vi "example_GProgramUploadFile.vi"() -> ()   [LabVIEW 2020]
uses:
  <vilib>/Galil/resources/gclib/gclib.lvlib
  <vilib>/Galil/resources/gclibo/gclibo.lvlib
panel:
  in  "File Location":string="C:\\Program Files\\National Instruments\\LabVIEW 2020\\vi.lib\\Galil\\examples\\vi_examples\\example_files\\dmc_upload.dmc"
  in  "Program":string="#test\nMG TIME\nEN"
  out "Error Out":errorcluster
  in  "IP Address":string="192.168.1.77"
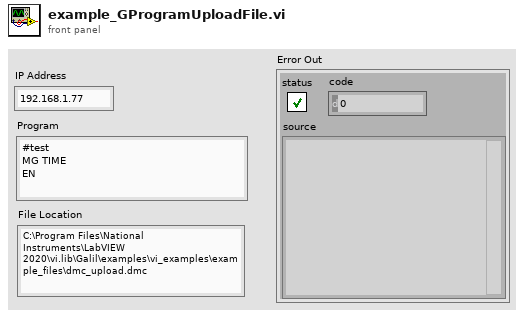
[diagram p1: front panel]
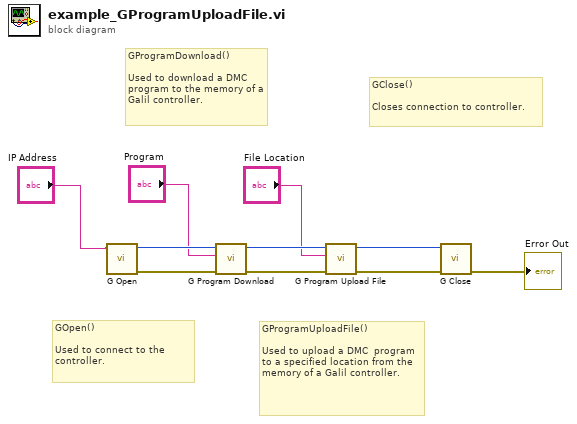
[diagram p0: block diagram]
diagram:
  # "GClose()\n\nCloses connection to controller."
  # "GProgramUploadFile()\n\nUsed to upload a DMC  program to a specified location from the memory of a Galil controller."
  # "GProgramDownload()\n\nUsed to download a DMC  program to the memory of a Galil controller."
  # "GOpen()\n\nUsed to connect to the controller."
  n1 = call <vilib>:"G Open.vi"("address"="IP Address") -> ("error out"=w4:errorcluster, "g out"=w6:u64)  [unwired: 8 in]
  n2 = call <vilib>:"G Program Download.vi"("error in (no error)"=w4, "program"="Program", "g"=w6) -> ("error out"=w3:errorcluster, "g out"=w2:u64)  [unwired: 7 in]
  n3 = call <vilib>:"G Program Upload File.vi"("error in (no error)"=w3, "file_path"="File Location", "g"=w2) -> ("error out"=w9:errorcluster, "g out"=w10:u64)  [unwired: 6 in]
  n4 = call <vilib>:"G Close.vi"("error in (no error)"=w9, "g"=w10) -> ("error out"=→"Error Out":errorcluster)  [unwired: 9 in]
